vi "HXGetCaptionName.vi"(1 "stateInfoUSIConnect out":T1) -> (0 "String":string)   [LabVIEW 2017]
uses:
  <vilib>/Platform/storage/lvStorage.llb/_stateInfoWriteProps.ctl
  <vilib>/Platform/storage/lvStorage.llb/dataStorageParams.ctl
  <vilib>/Platform/storage/lvStorage.llb/_selectedProp.ctl
  <vilib>/Platform/storage/lvStorage.llb/dataModel.ctl
  <vilib>/Platform/storage/Storage.llb/usiTypeDef.ctl
  <vilib>/Platform/storage/Storage.llb/usiPropDef.ctl
  <vilib>/express/express shared/ex_EditUserDefinedProperties/usiDataType.ctl
  <vilib>/Platform/storage/Storage.llb/specialProperties.ctl
  <vilib>/Platform/storage/Storage.llb/usiOverwriteOptions.ctl
  <vilib>/Platform/storage/lvStorage.llb/TerminalDef.ctl
  <vilib>/Platform/storage/lvStorage.llb/_TerminalStyle.ctl
  <vilib>/Utility/XNodeSupport.llb/XRect32.ctl
  <vilib>/Platform/storage/Storage.llb/usiSequenceRepresentation.ctl
  <vilib>/Platform/storage/lvStorage.llb/channelType.ctl
  <vilib>/Platform/storage/lvStorage.llb/_dataTerminals.ctl
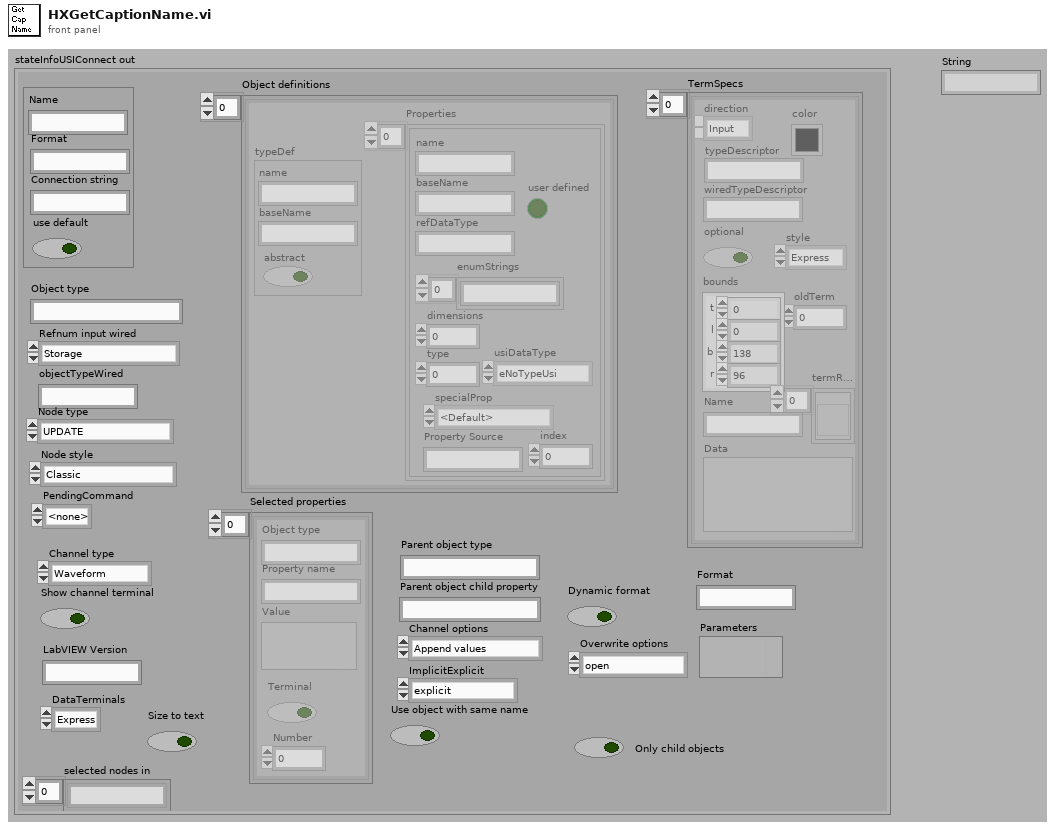
[diagram p1: front panel]
types:
  T1 = typedef "_stateInfoWriteProps.ctl" = cluster{"Data storage parameters":T2, "Object type":string, "Selected properties":T3[], "Object definitions":T4[], "Refnum input wired":enum16{"Storage", "Generic object", "Typed object", "<none>"}, "Parent object type":string, "Parent object child property":string, "Channel options":T9, "PendingCommand":enum16{"<none>", "SelPopUp", "Init"}, "Node style":enum16{"Classic", "Express"}, "Only child objects":bool, "TermSpecs":T10[], "objectTypeWired":string, "Dynamic format":bool, "Overwrite options":enum16{"open", "open or create", "create or replace", "create", "open (read only)"}, "Parameters":variant, "Format":string, "Node type":enum16{"UPDATE", "READ", "QUERY", "CREATE CHILD", "CREATE", "CONNECT", "DISCONNECT"}, "ImplicitExplicit":T13, "Channel type":T14, "Use object with same name":bool, "Show channel terminal":bool, "LabVIEW Version":string, "DataTerminals":T15, "Size to text":bool, "selected nodes in":string[]}
  T2 = typedef "dataStorageParams.ctl" = cluster{"Name":string, "Format":string, "Connection string":string, "use default":bool}
  T3 = typedef "_selectedProp.ctl" = cluster{"Object type":string, "Property name":string, "Value":variant, "Terminal":bool, "Number":i32}
  T4 = typedef "dataModel.ctl" = cluster{"typeDef":T5, "Properties":T6[]}
  T5 = typedef "usiTypeDef.ctl" = cluster{"name":string, "baseName":string, "abstract":bool}
  T6 = typedef "usiPropDef.ctl" = cluster{"name":string, "baseName":string, "refDataType":string, "dimensions":i32, "type":i32, "user defined":bool, "enumStrings":string[], "usiDataType":T7, "specialProp":T8, "Property Source":string, "index":i32}
  T7 = typedef "usiDataType.ctl" = enum16{"eNoTypeUsi", "eInt8Usi", "eInt16Usi", "eInt32Usi", "eInt64Usi", "eUInt8Usi", "eUInt16Usi", "eUInt32Usi", "eUInt64Usi", "eFloat32Usi", "eFloat64Usi", "- 0", "- 1", "- 2", "- 3", "- 4", "- 5", "- 6", "- 7", "- 8", "- 9", "eString8Usi", "eString16Usi", "eStringUsi", "eEnumUsi", "- 10", "- 11", "- 12", "- 13", "- 14", "eTimeUsi", "- 15", "- 16", "- 17", "- 18", "- 19", "- 20", "- 21", "- 22", "- 23", "eInstanceUsi", "eStoreUsi"}
  T8 = typedef "specialProperties.ctl" = enum16{"<Default>", "Channel Values", "AppendReplace", "ChannelFlags", "ValueFlags", "ImplicitExplicit", "InsertIndex", "ValuesCount", "ComparisonOperator", "Cluster", "DAQmx Channel"}
  T9 = typedef "usiOverwriteOptions.ctl" = enum16{"Append values", "Replace values at index", "Replace all values", "Append if timeline aligns"}
  T10 = typedef "TerminalDef.ctl" = cluster{"direction":enum16{"Input", "Output"}, "typeDescriptor":string, "color":u32, "oldTerm":i32, "style":T11, "optional":bool, "bounds":T12, "termRefs":refnum<vi>[], "Name":string, "Data":variant, "wiredTypeDescriptor":string}
  T11 = typedef "_TerminalStyle.ctl" = enum16{"Express", "Collapsed", "Internal"}
  T12 = typedef "XRect32.ctl" = cluster{"t":i32, "l":i32, "b":i32, "r":i32}
  T13 = typedef "usiSequenceRepresentation.ctl" = enum16{"explicit", "implicit"}
  T14 = typedef "channelType.ctl" = enum16{"Waveform", "Array of Double", "Array of String", "DDT", "Array of UInt8", "Array of Int16", "Array of Int32", "Array of Single", "Array of DateTime", "Array of Waveform", "none", "DateTime", "String", "Double", "Single", "UInt8", "Int16", "Int32"}
  T15 = typedef "_dataTerminals.ctl" = enum16{"Express", "Cluster"}
  T16 = enum16{"UPDATE", "READ", "QUERY", "CREATE CHILD", "CREATE", "CONNECT", "DISCONNECT"}
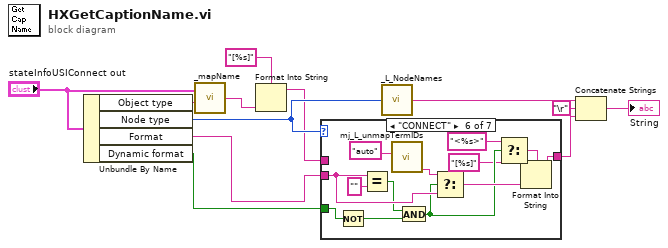
[diagram p0: block diagram]
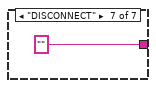
[diagram p7: hidden frame]
diagram:
  n1 = Unbundle By Name("stateInfoUSIConnect out") -> ("Object type"=w3:string, "Node type"=w8:T16, "Format"=w7:string, "Dynamic format"=w1:bool)
  n2 = call <vilib>:"_mapName.vi"("Object type"=w3, "stateInfo in"="stateInfoUSIConnect out") -> ("Object type"=w6:string)
  n3 = Format Into String(format string="[%s]", w6) -> (resulting string=w5:string)  [unwired: 2 in, 1 out]
  n4 = case shown="\"CONNECT\"" w8 {
    tunnel: w5 -> [w13 w14 w15 w16 w17 _ _]
    tunnel: [w13 w14 w15 w16 w17 w30 ""] -> w12
    tunnel: w7 -> [_ _ _ _ _ w28 _]
    tunnel: w1 -> [_ _ _ _ _ w25 _]
    frame "READ" {
    }
    frame "QUERY" {
    }
    frame "UPDATE" {
    }
    frame "CREATE CHILD" {
    }
    frame "CREATE" {
    }
    frame "CONNECT" {
      n5 = Not(x=w25) -> (.not. x?=w24:bool)
      n6 = Equal?(x=w28, y="") -> (x = y?=w26:bool)
      n7 = call <vilib>:"mj_L_unmapTermIDs.vi"("DNL_Name"="auto" ("t")) -> ("DNL_DisplayName"=w18:string)  [unwired: 6 in, 2 out]
      n8 = And(x=w26, y=w24) -> (x .and. y?=w23:bool)
      n9 = Select(t=w18, s=w23, f=w28) -> (s? t:f=w27:string)
      n10 = Select(t="<%s>" ("format string"), s=w23, f="[%s]" ("format string")) -> (s? t:f=w20:string)
      n11 = Format Into String(format string=w20, w27) -> (resulting string=w30:string)  [unwired: 2 in, 1 out]
    }
    frame "DISCONNECT" {
    }
  }
  n12 = call <vilib>:"_L_NodeNames.vi"("DNL_NodeType"=w8) -> ("DNL_NodeName"=w9:string)
  n13 = Concatenate Strings(w9, "\r", w12) -> (→"String":string)
